vi "Write Data Type Views.vi"(6 "Popup Title":string, 7 "Data Type Views":refnum<class "IAttribute Data Type View.lvclass">[](array[class]), 11 "ITest Executive Builder Dialog in":refnum<class "ITest Executive Builder Dialog.lvclass">) -> (3 "ITest Executive Builder Dialog out":refnum<class "ITest Executive Builder Dialog.lvclass">)   [LabVIEW 2017, in "ITest Executive Builder Dialog.lvclass"]
uses:
  ITest Executive Builder Dialog.lvclass
  <vilib>/gpm_packages/@cs/popup-viewmanager/Source/Popup ViewManager/Popup ViewManager.lvclass
  IAttribute Data Type View/IAttribute Data Type View.lvclass
  C:/Users/jonmc/Documents/Git/Test Executive Builder/gpm_packages/@cs/mva-framework/Source/Framework/IViewable/IViewable/IViewable.lvclass
  C:/Users/jonmc/Documents/Git/Test Executive Builder/gpm_packages/@cs/popup-viewmanager/Source/Popup ViewManager/Popup ViewManager.lvclass
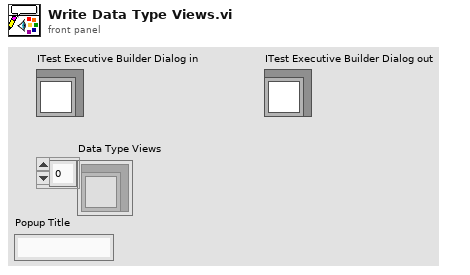
[diagram p1: front panel]
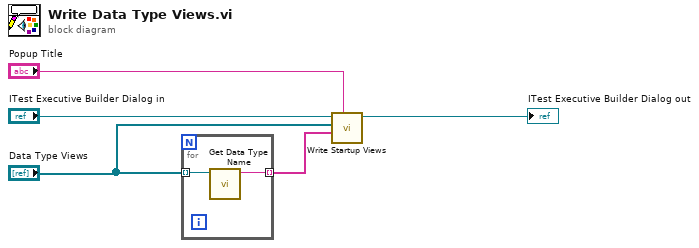
[diagram p0: block diagram]
diagram:
  n1 = for {
    tunnel: "Data Type Views" -> [w7] mode=indexing
    tunnel: [w6] -> w2 mode=indexing
    n2 = call-dynamic "Get Data Type Name.vi"("IAttribute Data Type View in"=w7) -> ("Data Type Name"=w6:string)  [unwired: 10 in]
  }
  n3 = call <vilib>:"Write Startup Views.vi"("Popup Title"="Popup Title", "View Labels (optional)"=w2, "Viewables"="Data Type Views", "Popup ViewManager in"="ITest Executive Builder Dialog in") -> ("Popup ViewManager out"=→"ITest Executive Builder Dialog out":refnum<class "ITest Executive Builder Dialog.lvclass">)  [unwired: 7 in]
